vi "Shutter Control.vi"(8 "Laser Shutter":T1(radio), 9 "error in":errorcluster, 11 "Camera Shutter":bool) -> (0 "error out":errorcluster)   [LabVIEW 2014]
uses:
  Shutter SubVis/Global Shutter Variables - SubVI.vi
panel:
  out "Current Wheel Position":string
  in  "Wheel Speed":u8=1 min=1 max=7 step=1
  in  "stop":bool
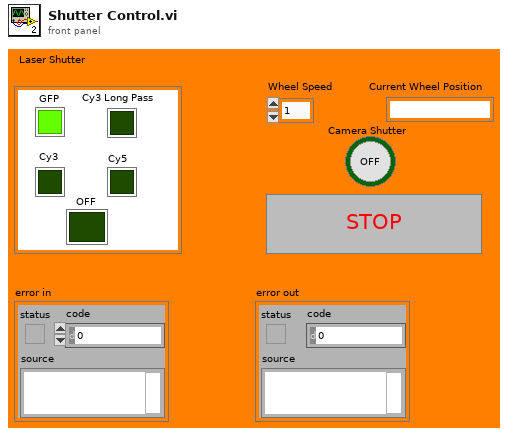
[diagram p1: front panel]
types:
  T1 = enum32{"GFP", "Cy3 Long Pass", "Cy3", "Cy5", "OFF"}
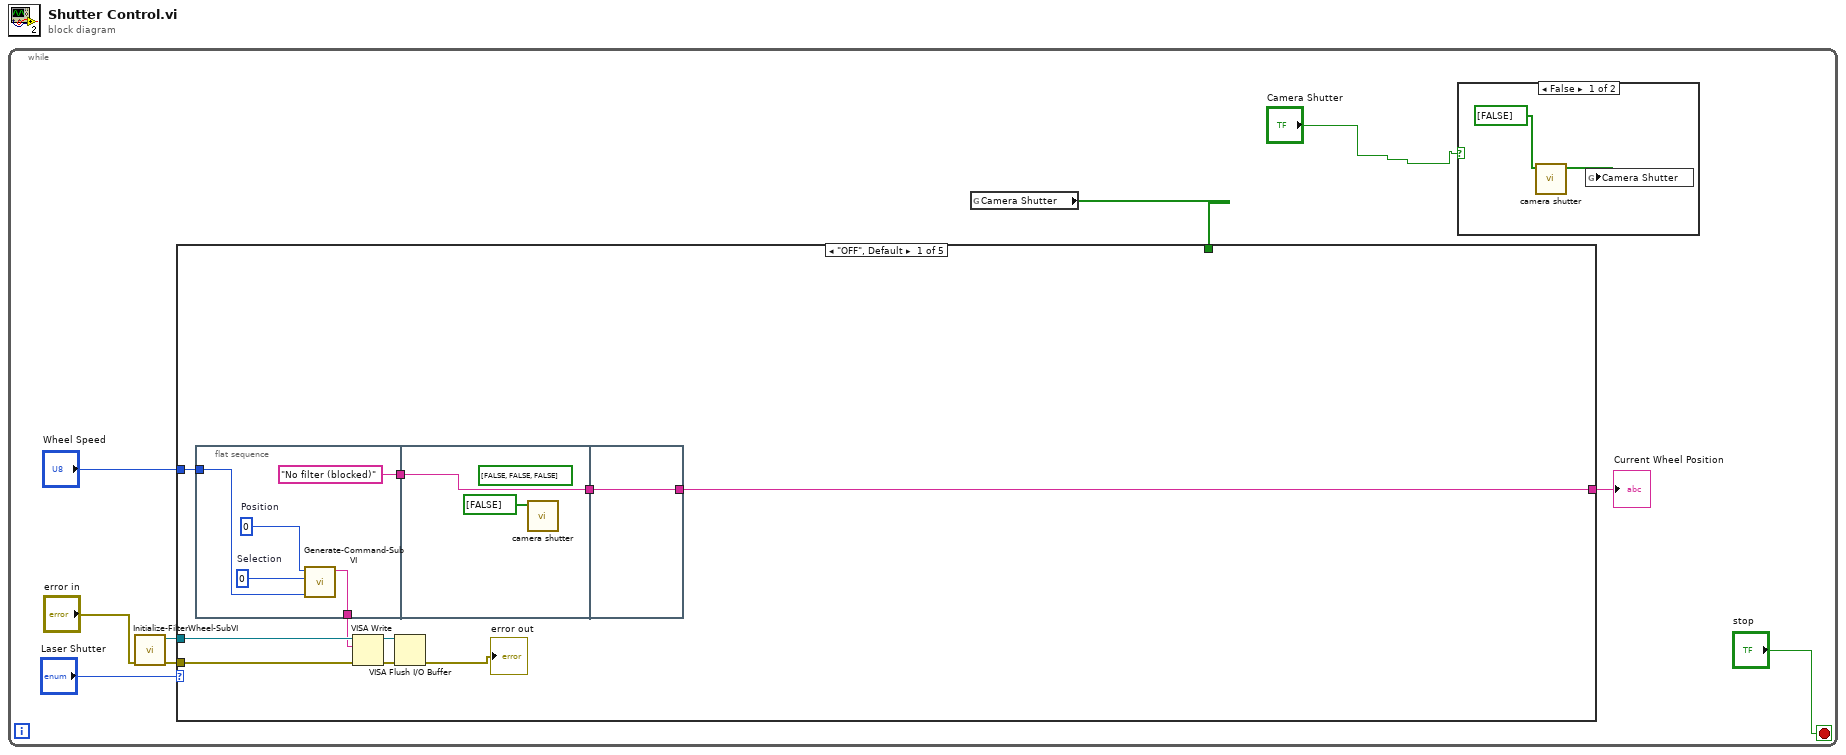
[diagram p0: block diagram]
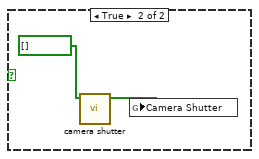
[diagram p2: hidden frame]
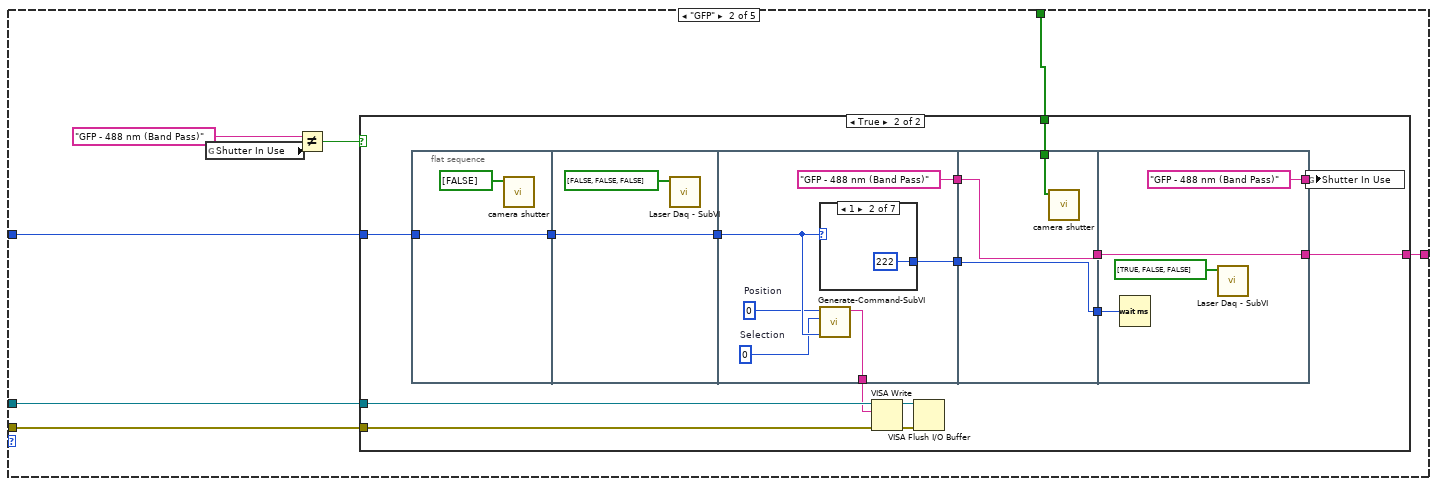
[diagram p3: hidden frame]
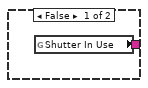
[diagram p4: hidden frame]
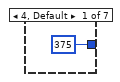
[diagram p5: hidden frame]
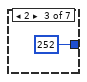
[diagram p6: hidden frame]
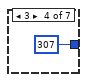
[diagram p7: hidden frame]
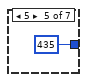
[diagram p8: hidden frame]
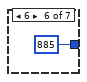
[diagram p9: hidden frame]
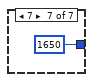
[diagram p10: hidden frame]
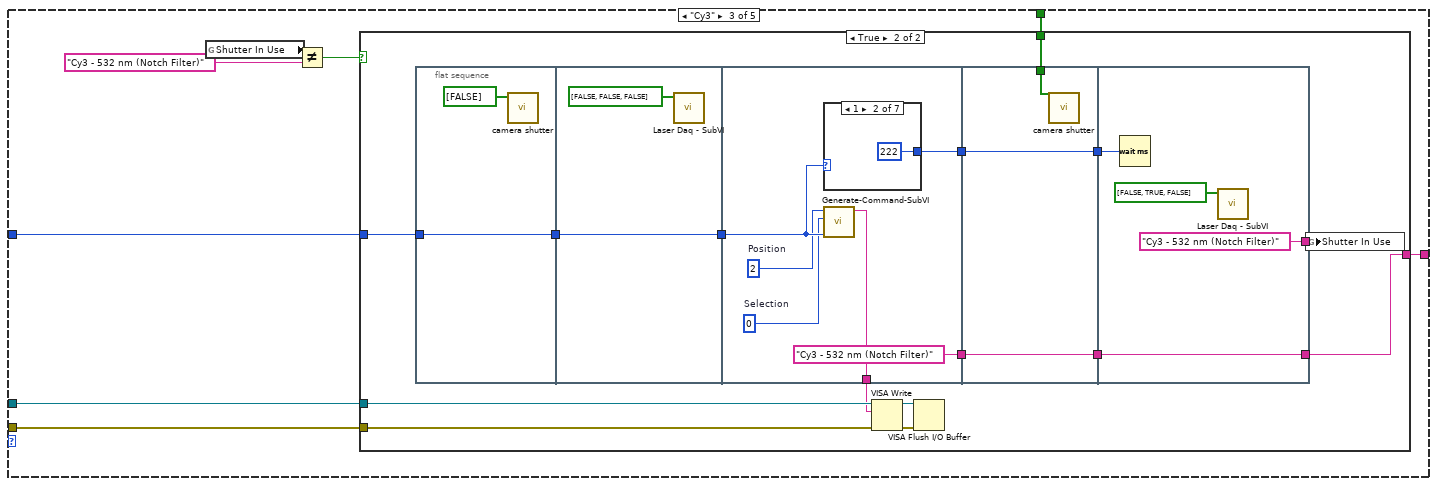
[diagram p11: hidden frame]
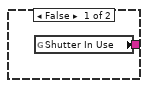
[diagram p12: hidden frame]
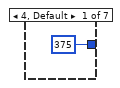
[diagram p13: hidden frame]
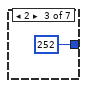
[diagram p14: hidden frame]
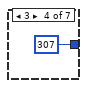
[diagram p15: hidden frame]
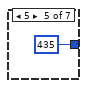
[diagram p16: hidden frame]
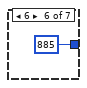
[diagram p17: hidden frame]
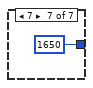
[diagram p18: hidden frame]
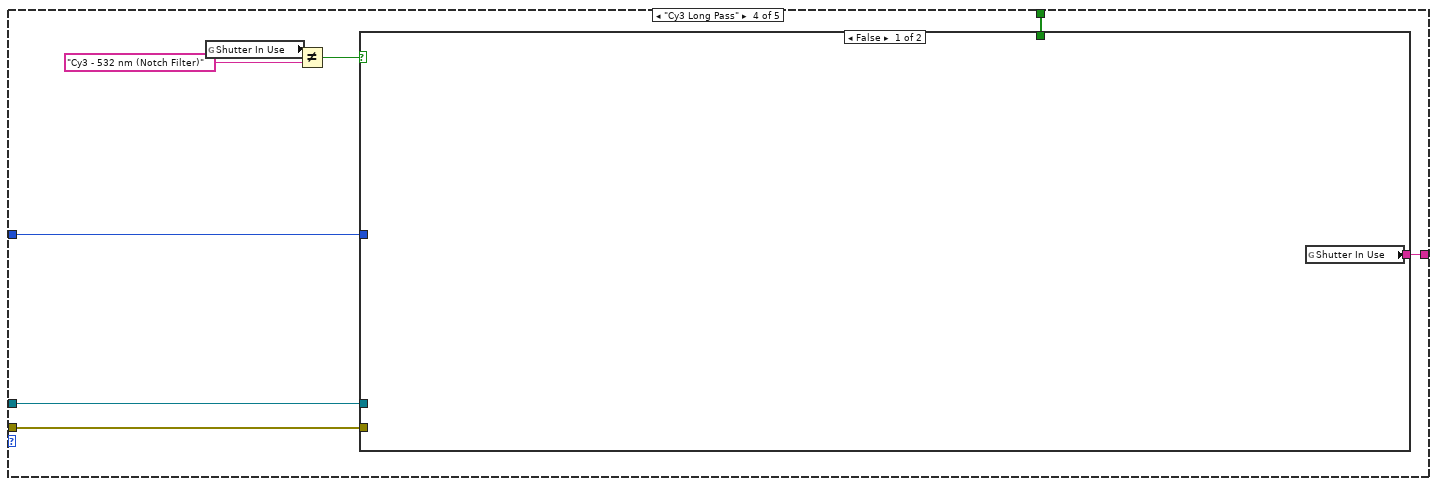
[diagram p19: hidden frame]
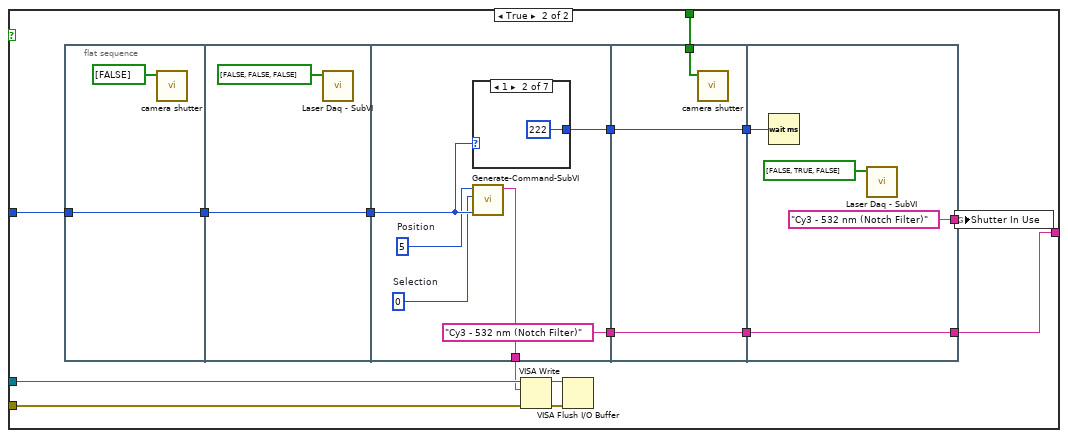
[diagram p20: hidden frame]
diagram:
  n1 = while {
    stop <- "stop" stop-if-true
    n2 = call "Initialize-FilterWheel-SubVI.vi"("error in"="error in") -> ("VISA resource name out"=w6:refnum<visa-resource-name>, "error out"=w5:errorcluster)  [unwired: 8 in]
    n3 = global read "Global Shutter Variables - SubVI.vi" "Camera Shutter"() -> (w3:bool[])
    n4 = case shown="\"OFF\", Default" "Laser Shutter" {
      tunnel: "Wheel Speed" -> [w23 w39 w87 w135 w183]
      tunnel: w6 -> [w20 w38 w86 w134 w182]
      tunnel: w5 -> [w19 w32 w85 w133 w181]
      tunnel: [w17 w37 w84 w132 w180] -> w4
      tunnel: w3 -> [_ w33 w80 w128 w176]
      frame "OFF", Default {
        n5 = flat-sequence {
          tunnel: w23 -> [w28]
          tunnel: [w25] -> w18
          tunnel: ["No filter (blocked)"] -> w16
          tunnel: w16 -> [w30]
          tunnel: [w30] -> w15
          tunnel: [w31] -> w17
          tunnel: w15 -> [w31]
          frame #0 {
            w26 = 0  # Selection
            w27 = 0  # Position
            n6 = call "Generate-Command-SubVI.vi"("Wheel Speed"=w28, "Wheel Selection"=w26, "Wheel Position"=w27) -> ("type"=w25:string)  [unwired: 8 in]
          }
          frame #1 {
            (unwired) bool[] [FALSE, FALSE, FALSE]
            n7 = call "camera shutter.vi"("Array"=bool[] [FALSE]) -> ()  [unwired: 10 in, 1 out]
          }
          frame #2 {
          }
        }
        n8 = VISA Write(VISA resource name=w20, write buffer=w18, error in (no error)=w19) -> (VISA resource name out=w21:refnum<visa-resource-name>, error out=w22:errorcluster)  [unwired: 1 out]
        n9 = VISA Flush I/O Buffer(VISA resource name=w21, error in (no error)=w22) -> (error out=→"error out":errorcluster)  [unwired: 1 in, 1 out]
      }
      frame "GFP" {
        n10 = global read "Global Shutter Variables - SubVI.vi" "Shutter In Use"() -> (w35:string)
        n11 = Not Equal?(x="GFP - 488 nm (Band Pass)", y=w35) -> (x != y?=w34:bool)
        n12 = case shown="True" w34 {
          tunnel: w39 -> [_ w50]
          tunnel: w38 -> [_ w47]
          tunnel: w32 -> [_ w46]
          tunnel: [w40 w44] -> w37
          tunnel: w33 -> [_ w41]
          frame False {
            n13 = global read "Global Shutter Variables - SubVI.vi" "Shutter In Use"() -> (w40:string)
          }
          frame True {
            n14 = flat-sequence {
              tunnel: w50 -> [w57]
              tunnel: [w57] -> w42
              tunnel: [w59] -> w55
              tunnel: w42 -> [w59]
              tunnel: [w62] -> w54
              tunnel: [w61] -> w45
              tunnel: ["GFP - 488 nm (Band Pass)"] -> w53
              tunnel: w55 -> [w65]
              tunnel: w54 -> [w74]
              tunnel: w53 -> [w75]
              tunnel: [w75] -> w52
              tunnel: [w74] -> w51
              tunnel: w41 -> [w73]
              tunnel: [w77] -> w44
              tunnel: w52 -> [w77]
              tunnel: w51 -> [w79]
              tunnel: ["GFP - 488 nm (Band Pass)"] -> w43
              frame #0 {
                n15 = call "camera shutter.vi"("Array"=bool[] [FALSE]) -> ()  [unwired: 10 in, 1 out]
              }
              frame #1 {
                n16 = call "Laser Daq - SubVI.vi"("Array"=bool[] [FALSE, FALSE, FALSE]) -> ()  [unwired: 11 in]
              }
              frame #2 {
                w63 = 0  # Selection
                w64 = 0  # Position
                n17 = case shown="1" w65 {
                  tunnel: [375 222 252 307 435 885 1650] -> w62
                  frame 4, Default {
                  }
                  frame 1 {
                  }
                  frame 2 {
                  }
                  frame 3 {
                  }
                  frame 5 {
                  }
                  frame 6 {
                  }
                  frame 7 {
                  }
                }
                n18 = call "Generate-Command-SubVI.vi"("Wheel Speed"=w65, "Wheel Selection"=w63, "Wheel Position"=w64) -> ("type"=w61:string)  [unwired: 8 in]
              }
              frame #3 {
                n19 = call "camera shutter.vi"("Array"=w73) -> ()  [unwired: 10 in, 1 out]
              }
              frame #4 {
                n20 = Wait (ms)(milliseconds to wait=w79) -> ()  [unwired: 1 out]
                n21 = call "Laser Daq - SubVI.vi"("Array"=bool[] [TRUE, FALSE, FALSE]) -> ()  [unwired: 11 in]
              }
            }
            n22 = VISA Write(VISA resource name=w47, write buffer=w45, error in (no error)=w46) -> (VISA resource name out=w49:refnum<visa-resource-name>, error out=w48:errorcluster)  [unwired: 1 out]
            n23 = VISA Flush I/O Buffer(VISA resource name=w49, error in (no error)=w48) -> ()  [unwired: 1 in, 2 out]
            n24 = global write "Global Shutter Variables - SubVI.vi" "Shutter In Use"(w43) -> ()
          }
        }
      }
      frame "Cy3" {
        n25 = global read "Global Shutter Variables - SubVI.vi" "Shutter In Use"() -> (w82:string)
        n26 = Not Equal?(x=w82, y="Cy3 - 532 nm (Notch Filter)") -> (x != y?=w81:bool)
        n27 = case shown="True" w81 {
          tunnel: w87 -> [_ w102]
          tunnel: w86 -> [_ w99]
          tunnel: w85 -> [_ w98]
          tunnel: [w88 w96] -> w84
          tunnel: w80 -> [_ w89]
          frame False {
            n28 = global read "Global Shutter Variables - SubVI.vi" "Shutter In Use"() -> (w88:string)
          }
          frame True {
            n29 = flat-sequence {
              tunnel: w102 -> [w105]
              tunnel: [w105] -> w90
              tunnel: [w107] -> w103
              tunnel: w90 -> [w107]
              tunnel: [w110] -> w94
              tunnel: [w109] -> w97
              tunnel: ["Cy3 - 532 nm (Notch Filter)"] -> w92
              tunnel: w103 -> [w113]
              tunnel: w94 -> [w123]
              tunnel: [w123] -> w93
              tunnel: w92 -> [w122]
              tunnel: [w122] -> w91
              tunnel: w89 -> [w121]
              tunnel: w93 -> [w127]
              tunnel: [w126] -> w96
              tunnel: w91 -> [w126]
              tunnel: ["Cy3 - 532 nm (Notch Filter)"] -> w95
              frame #0 {
                n30 = call "camera shutter.vi"("Array"=bool[] [FALSE]) -> ()  [unwired: 10 in, 1 out]
              }
              frame #1 {
                n31 = call "Laser Daq - SubVI.vi"("Array"=bool[] [FALSE, FALSE, FALSE]) -> ()  [unwired: 11 in]
              }
              frame #2 {
                w111 = 0  # Selection
                w112 = 2  # Position
                n32 = case shown="1" w113 {
                  tunnel: [375 222 252 307 435 885 1650] -> w110
                  frame 4, Default {
                  }
                  frame 1 {
                  }
                  frame 2 {
                  }
                  frame 3 {
                  }
                  frame 5 {
                  }
                  frame 6 {
                  }
                  frame 7 {
                  }
                }
                n33 = call "Generate-Command-SubVI.vi"("Wheel Speed"=w113, "Wheel Selection"=w111, "Wheel Position"=w112) -> ("type"=w109:string)  [unwired: 8 in]
              }
              frame #3 {
                n34 = call "camera shutter.vi"("Array"=w121) -> ()  [unwired: 10 in, 1 out]
              }
              frame #4 {
                n35 = Wait (ms)(milliseconds to wait=w127) -> ()  [unwired: 1 out]
                n36 = call "Laser Daq - SubVI.vi"("Array"=bool[] [FALSE, TRUE, FALSE]) -> ()  [unwired: 11 in]
              }
            }
            n37 = VISA Write(VISA resource name=w99, write buffer=w97, error in (no error)=w98) -> (VISA resource name out=w101:refnum<visa-resource-name>, error out=w100:errorcluster)  [unwired: 1 out]
            n38 = VISA Flush I/O Buffer(VISA resource name=w101, error in (no error)=w100) -> ()  [unwired: 1 in, 2 out]
            n39 = global write "Global Shutter Variables - SubVI.vi" "Shutter In Use"(w95) -> ()
          }
        }
      }
      frame "Cy3 Long Pass" {
        n40 = global read "Global Shutter Variables - SubVI.vi" "Shutter In Use"() -> (w131:string)
        n41 = Not Equal?(x=w131, y="Cy3 - 532 nm (Notch Filter)") -> (x != y?=w129:bool)
        n42 = case shown="False" w129 {
          tunnel: w135 -> [_ w150]
          tunnel: w134 -> [_ w147]
          tunnel: w133 -> [_ w146]
          tunnel: [w136 w144] -> w132
          tunnel: w128 -> [_ w137]
          frame False {
            n43 = global read "Global Shutter Variables - SubVI.vi" "Shutter In Use"() -> (w136:string)
          }
          frame True {
            n44 = flat-sequence {
              tunnel: w150 -> [w153]
              tunnel: [w153] -> w142
              tunnel: [w155] -> w151
              tunnel: w142 -> [w155]
              tunnel: [w158] -> w141
              tunnel: [w157] -> w145
              tunnel: ["Cy3 - 532 nm (Notch Filter)"] -> w139
              tunnel: w151 -> [w161]
              tunnel: w141 -> [w171]
              tunnel: [w171] -> w140
              tunnel: w139 -> [w170]
              tunnel: [w170] -> w138
              tunnel: w137 -> [w169]
              tunnel: w140 -> [w175]
              tunnel: [w174] -> w144
              tunnel: w138 -> [w174]
              tunnel: ["Cy3 - 532 nm (Notch Filter)"] -> w143
              frame #0 {
                n45 = call "camera shutter.vi"("Array"=bool[] [FALSE]) -> ()  [unwired: 10 in, 1 out]
              }
              frame #1 {
                n46 = call "Laser Daq - SubVI.vi"("Array"=bool[] [FALSE, FALSE, FALSE]) -> ()  [unwired: 11 in]
              }
              frame #2 {
                w159 = 0  # Selection
                w160 = 5  # Position
                n47 = case shown="1" w161 {
                  tunnel: [375 222 252 307 435 885 1650] -> w158
                  frame 4, Default {
                  }
                  frame 1 {
                  }
                  frame 2 {
                  }
                  frame 3 {
                  }
                  frame 5 {
                  }
                  frame 6 {
                  }
                  frame 7 {
                  }
                }
                n48 = call "Generate-Command-SubVI.vi"("Wheel Speed"=w161, "Wheel Selection"=w159, "Wheel Position"=w160) -> ("type"=w157:string)  [unwired: 8 in]
              }
              frame #3 {
                n49 = call "camera shutter.vi"("Array"=w169) -> ()  [unwired: 10 in, 1 out]
              }
              frame #4 {
                n50 = Wait (ms)(milliseconds to wait=w175) -> ()  [unwired: 1 out]
                n51 = call "Laser Daq - SubVI.vi"("Array"=bool[] [FALSE, TRUE, FALSE]) -> ()  [unwired: 11 in]
              }
            }
            n52 = VISA Write(VISA resource name=w147, write buffer=w145, error in (no error)=w146) -> (VISA resource name out=w149:refnum<visa-resource-name>, error out=w148:errorcluster)  [unwired: 1 out]
            n53 = VISA Flush I/O Buffer(VISA resource name=w149, error in (no error)=w148) -> ()  [unwired: 1 in, 2 out]
            n54 = global write "Global Shutter Variables - SubVI.vi" "Shutter In Use"(w143) -> ()
          }
        }
      }
      frame "Cy5" {
        n55 = global read "Global Shutter Variables - SubVI.vi" "Shutter In Use"() -> (w179:string)
        n56 = Not Equal?(x=w179, y="Cy5 - 637 (Notch Filter)") -> (x != y?=w177:bool)
        n57 = case shown="False" w177 {
          tunnel: w183 -> [_ w198]
          tunnel: w182 -> [_ w195]
          tunnel: w181 -> [_ w194]
          tunnel: [w184 w192] -> w180
          tunnel: w176 -> [_ w185]
          frame False {
            n58 = global read "Global Shutter Variables - SubVI.vi" "Shutter In Use"() -> (w184:string)
          }
          frame True {
            n59 = flat-sequence {
              tunnel: w198 -> [w201]
              tunnel: [w201] -> w190
              tunnel: [w203] -> w199
              tunnel: w190 -> [w203]
              tunnel: [w206] -> w189
              tunnel: [w205] -> w193
              tunnel: ["Cy5 - 637 (Notch Filter)"] -> w187
              tunnel: w199 -> [w209]
              tunnel: w189 -> [w219]
              tunnel: [w219] -> w188
              tunnel: w187 -> [w218]
              tunnel: [w218] -> w186
              tunnel: w185 -> [w217]
              tunnel: w188 -> [w223]
              tunnel: [w222] -> w192
              tunnel: w186 -> [w222]
              tunnel: ["Cy5 - 637 (Notch Filter)"] -> w191
              frame #0 {
                n60 = call "camera shutter.vi"("Array"=bool[] [FALSE]) -> ()  [unwired: 10 in, 1 out]
              }
              frame #1 {
                n61 = call "Laser Daq - SubVI.vi"("Array"=bool[] [FALSE, FALSE, FALSE]) -> ()  [unwired: 11 in]
              }
              frame #2 {
                w207 = 0  # Selection
                w208 = 7  # Position
                n62 = case shown="1" w209 {
                  tunnel: [375 222 252 307 435 885 1650] -> w206
                  frame 4, Default {
                  }
                  frame 1 {
                  }
                  frame 2 {
                  }
                  frame 3 {
                  }
                  frame 5 {
                  }
                  frame 6 {
                  }
                  frame 7 {
                  }
                }
                n63 = call "Generate-Command-SubVI.vi"("Wheel Speed"=w209, "Wheel Selection"=w207, "Wheel Position"=w208) -> ("type"=w205:string)  [unwired: 8 in]
              }
              frame #3 {
                n64 = call "camera shutter.vi"("Array"=w217) -> ()  [unwired: 10 in, 1 out]
              }
              frame #4 {
                n65 = Wait (ms)(milliseconds to wait=w223) -> ()  [unwired: 1 out]
                n66 = call "Laser Daq - SubVI.vi"("Array"=bool[] [FALSE, FALSE, TRUE]) -> ()  [unwired: 11 in]
              }
            }
            n67 = VISA Write(VISA resource name=w195, write buffer=w193, error in (no error)=w194) -> (VISA resource name out=w197:refnum<visa-resource-name>, error out=w196:errorcluster)  [unwired: 1 out]
            n68 = VISA Flush I/O Buffer(VISA resource name=w197, error in (no error)=w196) -> ()  [unwired: 1 in, 2 out]
            n69 = global write "Global Shutter Variables - SubVI.vi" "Shutter In Use"(w191) -> ()
          }
        }
      }
    }
    "Current Wheel Position" <- w4
    n70 = case shown="False" "Camera Shutter" {
      frame False {
        n71 = call "camera shutter.vi"("Array"=bool[] [FALSE]) -> ("Array 2"=w11:bool[])  [unwired: 10 in]
        n72 = global write "Global Shutter Variables - SubVI.vi" "Camera Shutter"(w11) -> ()
      }
      frame True {
        n73 = call "camera shutter.vi"("Array"=bool[] []) -> ("Array 2"=w13:bool[])  [unwired: 10 in]
        n74 = global write "Global Shutter Variables - SubVI.vi" "Camera Shutter"(w13) -> ()
      }
    }
  }
